vi "TDS RF Signal Output State.vi"(8 "error in (no error)":errorcluster, 9 "Output State":bool, 10 "Signal InstConfig":string, 11 "Address":string) -> (0 "error out":errorcluster)   [LabVIEW 2025, in "Interface Functions.lvlib"]
uses:
  Interface Functions.lvlib
panel:
  out "read buffer":string
  # "RF Signal Output State"
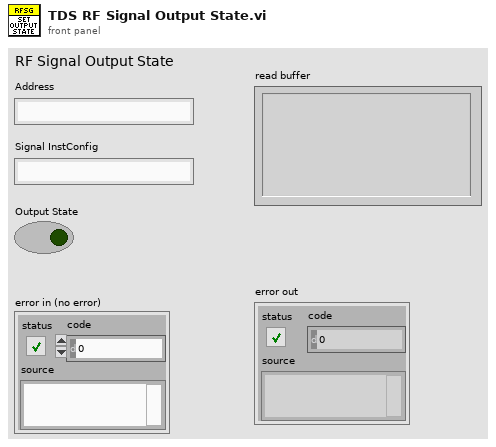
[diagram p1: front panel]
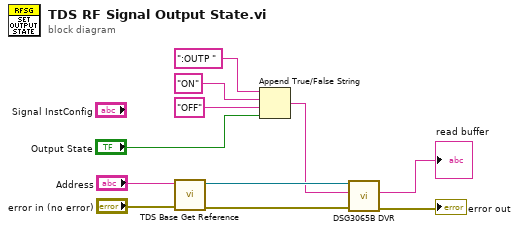
[diagram p0: block diagram]
diagram:
  n1 = call "TDS Base Get Reference.vi"("error in (no error)"="error in (no error)", "Address"="Address") -> ("error out"=w5:errorcluster, "Reference"=w3:refnum<visa-resource-name>)  [unwired: 8 in]
  n2 = Append True/False String(1:"Output State", 2:"OFF", 3:"ON", 4:":OUTP ") -> (0:w2:string)
  n3 = call "DSG3065B DVR.vi"("error in (no error)"=w5, "write buffer"=w2, "VISA resource name"=w3) -> ("error out"=→"error out":errorcluster, "read buffer"=→"read buffer":string)  [unwired: 7 in]
